vi "SCH.vi"(0 "System no.":i32=1 min=1 max=4 step=1, 2 "Axis name":string, 5 "error in":errorcluster) -> (19 "error out":errorcluster)   [LabVIEW 2020]
doc: "Set axis (channel) name. See system manual for further description. Run Define connected axes.vi after renaming axes. \n\nE-816: This command cannot be issued to a slave E-816. Changes must be written to non-volatile memory with WPA.vi. and do not take effect before the next power on or RST."
panel:
  # "Set axis (channel) name. Changes must be written to\nnon-volatile memory with WPA.vi and do not take\neffect before the next power on or RST. Run \n\"Define connected axes\" after renaming axes."
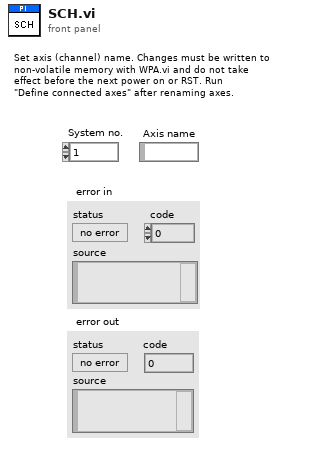
[diagram p1: front panel]
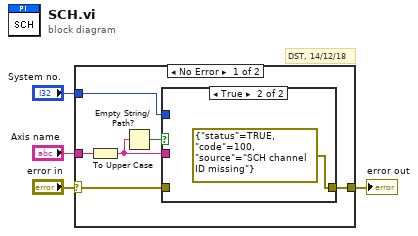
[diagram p0: block diagram]
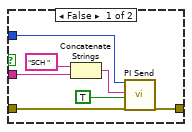
[diagram p2: hidden frame]
diagram:
  # "DST, 14/12/18"
  n1 = case shown="No Error" "error in" {
    selector: "error in" -> [w7 w19]
    tunnel: "Axis name" -> [w10 _]
    tunnel: "System no." -> [w9 _]
    tunnel: [w8 w19] -> w2
    frame No Error {
      n2 = To Upper Case(1:w10) -> (0:w6:string)
      n3 = Empty String/Path?(string/path=w6) -> (empty?=w5:bool)
      n4 = case shown="True" w5 {
        tunnel: w7 -> [w12 _]
        tunnel: w9 -> [w14 _]
        tunnel: [w13 errorcluster {"status"=TRUE, "code"=100, "source"="SCH channel ID missing"} ("error out")] -> w8
        tunnel: w6 -> [w11 _]
        frame False {
          n5 = Concatenate Strings("SCH ", w11) -> (w15:string)
          n6 = call "PI Send.vi"("System no."=w14, "String to send"=w15, "Attach termination char.?"=TRUE ("Attach Linefeed?"), "error in"=w12) -> ("error out"=w13:errorcluster)  [unwired: 2 in, 13 out]
        }
        frame True {
        }
      }
    }
    frame Error {
    }
  }
  "error out" <- w2
